vi "Find best matching frame.vi"(7 "Timelapse video is master":bool=TRUE, 9 "Frame number in master video":i32=1 min=1, 11 "Cam video frame numbers & locations":T1) -> (1 "Nearest available frame number in slave video":i64, 3 "Nearest frame position in Cam binary file":i64)   [LabVIEW 2017]
uses:
  Typedefs/Number of frames and locations cluster.ctl
  Globals/gl_Time series viewer globals.vi
  <vilib>/gmath/NI_Gmath.lvlib
panel:
  out "Nearest rel. time":i64
  in  "Timelapse video's frame numbers":i64[](array[numeric])
  out "Fractional index in slave video":dbl
  out "Range of slave video frame numbers":i64[](array[numeric])
  out "Range of master video frame numbers":i64[](array[numeric])
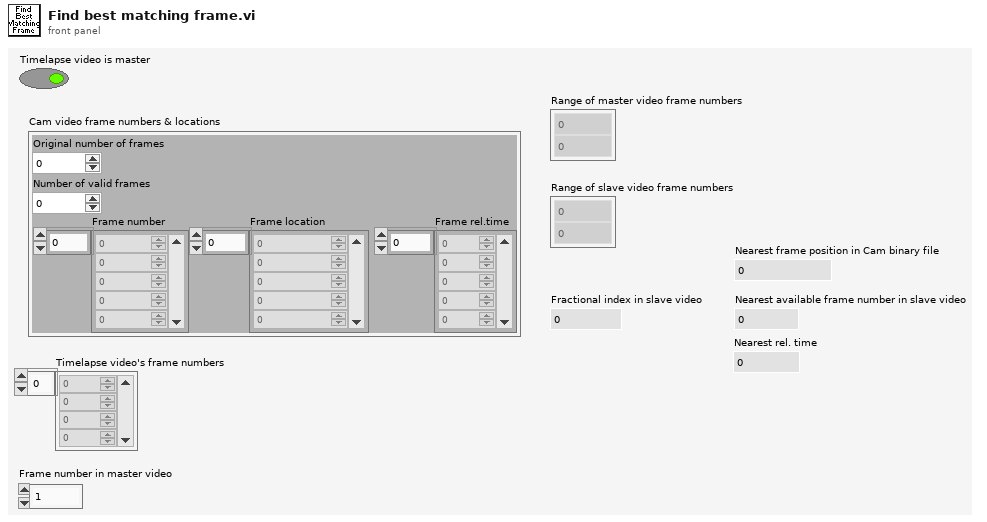
[diagram p1: front panel]
types:
  T1 = typedef "Number of frames and locations cluster.ctl" = cluster{"Original number of frames":i32, "Number of valid frames":i32, "Frame number":i64[], "Frame location":i64[], "Frame rel.time":i64[]}
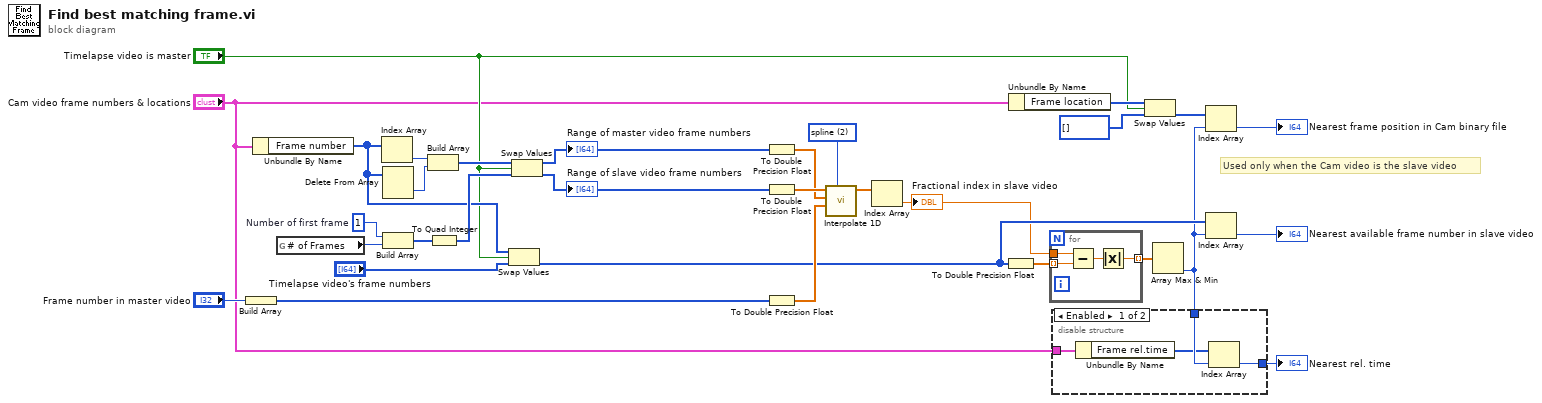
[diagram p0: block diagram]
diagram:
  w26 = 2 items=["nearest", "linear", "spline", "cubic Hermite", "Lagrange"] ("method")
  w29 = u32 1  # Number of first frame
  # "Used only when the Cam video is the slave video"
  n1 = Build Array("Frame number in master video") -> (w30:i32[])
  n2 = Unbundle By Name("Cam video frame numbers & locations") -> ("Frame number"=w16:i64[])
  n3 = global read "gl_Time series viewer globals.vi" "# of Frames"() -> (w27:u32)
  n4 = Index Array(array=w16) -> (element=w25:i64)  [unwired: 1 in]
  n5 = Delete From Array(array=w16) -> (deleted portion=w24:i64)  [unwired: 2 in, 1 out]
  n6 = Build Array(w29, w27) -> (w20:u32[])
  n7 = Build Array(w25, w24) -> (w21:i64[])
  n8 = To Quad Integer(1:w20) -> (0:w19:i64[])
  n9 = Swap Values(12:w16, 13:"Timelapse video is master", 14:"Timelapse video's frame numbers") -> (3:w13:i64[])  [unwired: 1 out]
  n10 = Swap Values(12:w21, 13:"Timelapse video is master", 14:w19) -> (1:w22:i64[], 3:w14:i64[])
  "Range of master video frame numbers" <- w22
  "Range of slave video frame numbers" <- w14
  n11 = To Double Precision Float(number=w22) -> (double precision float=w5:dbl[])
  n12 = To Double Precision Float(number=w14) -> (double precision float=w6:dbl[])
  n13 = To Double Precision Float(number=w30) -> (double precision float=w28:dbl[])
  n14 = call <vilib>:"Interpolate 1D.vi"("method"=w26, "xi"=w28, "X"=w5, "Y"=w6) -> ("yi"=w23:dbl[])  [unwired: 2 in, 5 out]
  n15 = Index Array(array=w23) -> (element=w12:dbl)  [unwired: 1 in]
  "Fractional index in slave video" <- w12
  n16 = To Double Precision Float(number=w13) -> (double precision float=w11:dbl[])
  n17 = Unbundle By Name("Cam video frame numbers & locations") -> ("Frame location"=w10:i64[])
  n18 = for {
    tunnel: w11 -> [w34] mode=indexing
    tunnel: w12 -> [w35]
    tunnel: [w32] -> w18 mode=indexing
    n19 = Subtract(x=w35, y=w34) -> (x-y=w33:dbl)
    n20 = Absolute Value(x=w33) -> (abs(x)=w32:dbl)
  }
  n21 = Swap Values(12:w10, 13:"Timelapse video is master", 14:i64[] [] ("Frame location")) -> (3:w8:i64[])  [unwired: 1 out]
  n22 = Array Max & Min(array=w18) -> (min index (indices)=w2:i32)  [unwired: 3 out]
  n23 = disable-structure shown="Enabled" {
    disable-tunnel: "Cam video frame numbers & locations" -> [w39 _]
    disable-tunnel: w2 -> [w38 _]
    disable-tunnel: [w36 _] -> w1
    frame Enabled {
      n24 = Unbundle By Name(w39) -> ("Frame rel.time"=w37:i64[])
      n25 = Index Array(array=w37, index=w38) -> (element=w36:i64)
    }
    frame Disabled {
    }
  }
  "Nearest rel. time" <- w1
  n26 = Index Array(array=w8, index=w2) -> (element=→"Nearest frame position in Cam binary file":i64)
  n27 = Index Array(array=w13, index=w2) -> (element=→"Nearest available frame number in slave video":i64)
